vi "Configure Battery Mode.vi"(7 "Channel":i32(ring)=1 items=["Channel 1"=1, "Channel 2"=2, "Channel 3"=3, "Channel 4"=4, "Channel 5"=5, "Channel 6"=6, "Channel 7"=7, "Channel 8"=8, "Channel 8"=9, "Channel 10"=10, "Channel 11"=11, "Channel 12"=12, "Channel 13"=13, "Channel 14"=14, "Channel 15"=15, "Channel 16"=16], 8 "error in":errorcluster, 10 "Battery Mode":u8(ring) items=["Charge", "Discharge"], 11 "VISA resource name":refnum<visa-resource-name>) -> (0 "error out":errorcluster, 3 "VISA resource name out":refnum<visa-resource-name>)   [LabVIEW 2020, in "IT-M3400.lvlib"]
doc: "Set the charging or discharging mode for the battery test.\n<b>Battery Mode</b>\n0:Charge\n1:Discharge"
uses:
  Desktop/Battery-Testing-Software - Shortcut.lnk/Drivers-IT-M3400/IT-M3400.lvlib
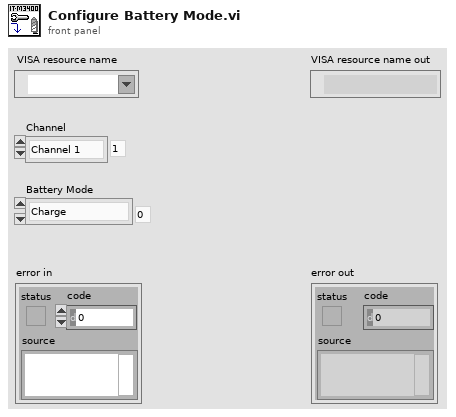
[diagram p1: front panel]
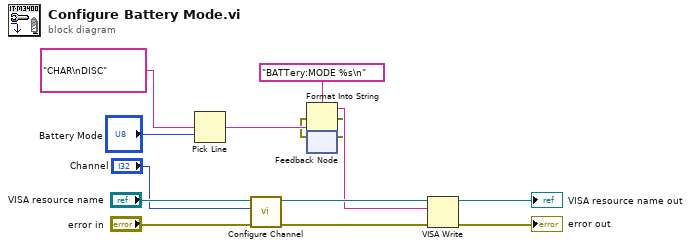
[diagram p0: block diagram]
diagram:
  n1 = Pick Line(multi-line string="CHAR\nDISC", line index="Battery Mode") -> (output string=w6:string)  [unwired: 1 in]
  n2 = call "Configure Channel.vi"("error in"="error in", "Channel"="Channel", "VISA resource name"="VISA resource name") -> ("error out"=w10:errorcluster, "VISA resource name out"=w11:refnum<visa-resource-name>)  [unwired: 7 in]
  n3 = feedback #1() -> (w3:errorcluster)  [unwired: 1 in]
  n4 = Format Into String(format string="BATTery:MODE %s\n", error in=w3, w6) -> (resulting string=w5:string, error out=w4:errorcluster)  [unwired: 1 in]
  n5 = feedback-in #1(w4) -> ()
  n6 = VISA Write(VISA resource name=w11, write buffer=w5, error in (no error)=w10) -> (VISA resource name out=→"VISA resource name out":refnum<visa-resource-name>, error out=→"error out":errorcluster)  [unwired: 1 out]
